vi "SMTP Email Alerts Messenger.vi"(0 "Notifier Name":string, 2 "Actions":T1, 7 "Recipient":string="Not An Address", 9 "Subject":string="No Subject", 11 "Body Text":string="No Message") -> ()   [LabVIEW 2016]
uses:
  SMTP Email Alerts Type Defs/SMTP Email Alerts Actions.ctl
  SMTP Email Alerts Type Defs/SMTP Email Alerts Notifier Type.ctl
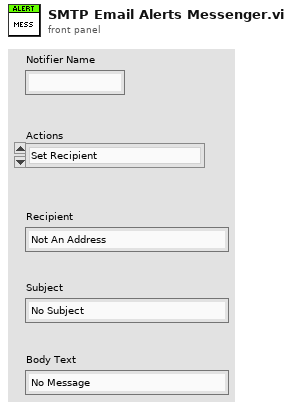
[diagram p1: front panel]
types:
  T1 = typedef "SMTP Email Alerts Actions.ctl" = enum16{"Set Recipient", "Send Message", "Quit"}
  T2 = typedef "SMTP Email Alerts Notifier Type.ctl" = cluster{"Actions":T1, "Recipient":string, "Subject":string, "Message":string}
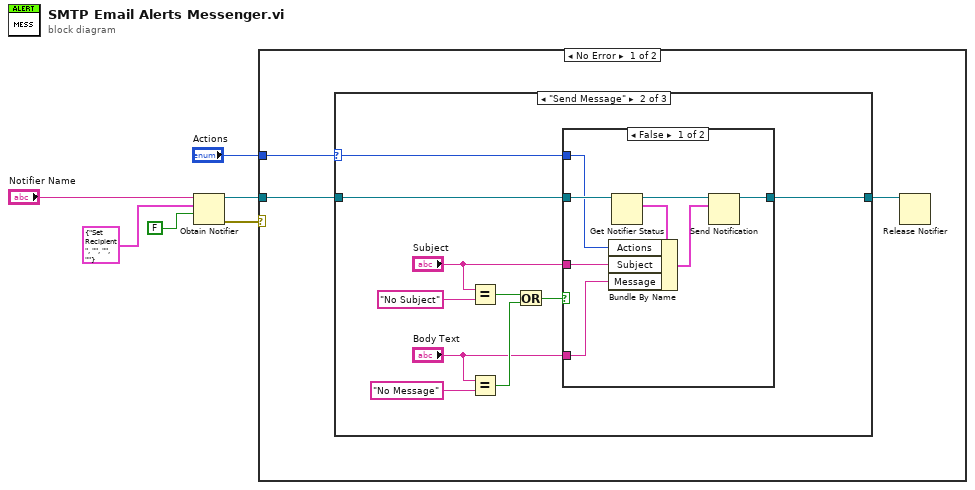
[diagram p0: block diagram]
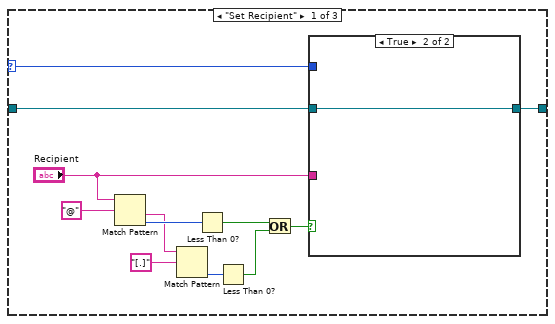
[diagram p2: hidden frame]
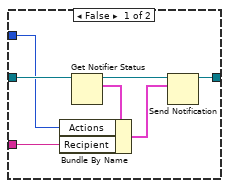
[diagram p3: hidden frame]
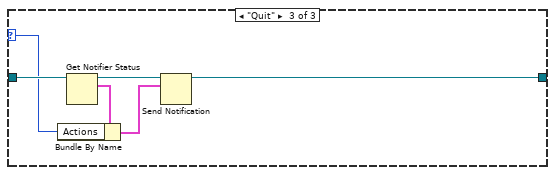
[diagram p5: hidden frame]
diagram:
  n1 = Obtain Notifier(name (unnamed)="Notifier Name", notification data type=T2 {"Actions"=enum."Set Recipient", "Recipient"="", "Subject"="", "Message"=""} ("Message Info"), create if not found? (T)=FALSE) -> (notifier out=w2:refnum<notifier>, error out=w3:errorcluster)  [unwired: 1 in, 1 out]
  n2 = case shown="No Error" w3 {
    tunnel: w2 -> [w8 _]
    tunnel: "Actions" -> [w9 _]
    frame No Error {
      n3 = case shown="\"Send Message\"" w9 {
        selector: w9 -> [w11 w33 w51]
        tunnel: w8 -> [w12 w34 w54]
        tunnel: [w10 w30 w49] -> w7
        frame "Set Recipient" {
          n4 = Match Pattern(string="Recipient", regular expression="@") -> (after substring=w15:string, offset past match=w18:i32)  [unwired: 1 in, 2 out]
          n5 = Match Pattern(string=w15, regular expression="[.]") -> (offset past match=w20:i32)  [unwired: 1 in, 3 out]
          n6 = Less Than 0?(x=w18) -> (x < 0?=w19:bool)
          n7 = Less Than 0?(x=w20) -> (x < 0?=w21:bool)
          n8 = Or(x=w19, y=w21) -> (x .or. y?=w14:bool)
          n9 = case shown="True" w14 {
            tunnel: "Recipient" -> [w24 _]
            tunnel: w12 -> [w25 w29]
            tunnel: w11 -> [w23 _]
            tunnel: [w22 w29] -> w10
            frame False {
              n10 = Get Notifier Status(notifier=w25) -> (notifier out=w27:refnum<notifier>, current notification=w28:T2)  [unwired: 1 in, 3 out]
              n11 = Bundle By Name(cluster=w28, "Actions"=w23, "Recipient"=w24) -> (w26:T2)
              n12 = Send Notification(notification=w26, notifier=w27) -> (notifier out=w22:refnum<notifier>)  [unwired: 1 in, 1 out]
            }
            frame True {
            }
          }
        }
        frame "Send Message" {
          n13 = Equal?(x="Subject", y="No Subject") -> (x = y?=w37:bool)
          n14 = Equal?(x="Body Text", y="No Message") -> (x = y?=w36:bool)
          n15 = Or(x=w37, y=w36) -> (x .or. y?=w35:bool)
          n16 = case shown="False" w35 {
            tunnel: w34 -> [w47 w48]
            tunnel: w33 -> [w44 _]
            tunnel: "Subject" -> [w42 _]
            tunnel: "Body Text" -> [w41 _]
            tunnel: [w40 w48] -> w30
            frame False {
              n17 = Get Notifier Status(notifier=w47) -> (notifier out=w46:refnum<notifier>, current notification=w45:T2)  [unwired: 1 in, 3 out]
              n18 = Bundle By Name(cluster=w45, "Actions"=w44, "Subject"=w42, "Message"=w41) -> (w43:T2)
              n19 = Send Notification(notification=w43, notifier=w46) -> (notifier out=w40:refnum<notifier>)  [unwired: 1 in, 1 out]
            }
            frame True {
            }
          }
        }
        frame "Quit" {
          n20 = Get Notifier Status(notifier=w54) -> (notifier out=w53:refnum<notifier>, current notification=w52:T2)  [unwired: 1 in, 3 out]
          n21 = Bundle By Name(cluster=w52, "Actions"=w51) -> (w50:T2)
          n22 = Send Notification(notification=w50, notifier=w53) -> (notifier out=w49:refnum<notifier>)  [unwired: 1 in, 1 out]
        }
      }
      n23 = Release Notifier(notifier=w7) -> ()  [unwired: 2 in, 3 out]
    }
    frame Error {
    }
  }
